vi "GenerateBurst.vi"(8 "error in (no error)":errorcluster, 9 "Burst mode":T1, 11 "reference in":refnum<class "niMmWave_Reciever.lvclass">) -> (0 "error out":errorcluster, 3 "reference out":refnum<class "niMmWave_Reciever.lvclass">)   [LabVIEW 2019, in "niMmWave_Reciever.lvclass"]
doc: "Generates single burst"
uses:
  niMmWave_Reciever.lvclass
  C:/Barkhausen mmWave radar/Development/LV/Barkhausen mmWave hardware control/Host/SubVIs/mmWave instrument_class/mmWave instrument.lvclass
  mmWave instrument_class/BurstMode.ctl
  mmWave HW Control/HW custom error.ctl
  mmWave instrument_class/Instrument state.ctl
  Low-level/TypeDefs/Direction.ctl
  mmWave HW Control/mmWave HW Control.lvlib
  mmWave instrument_class/mmWave instrument.lvclass
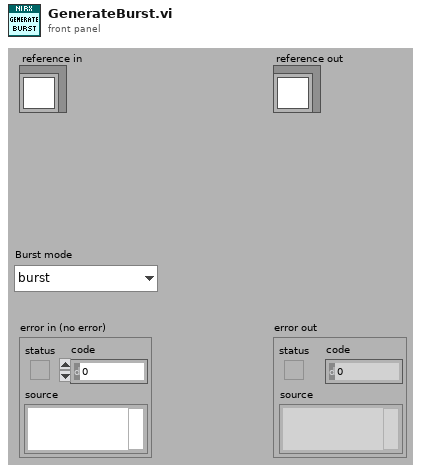
[diagram p1: front panel]
types:
  T1 = typedef "mmWave instrument.lvclass/BurstMode.ctl" = enum16{"burst", "continuous"}
  T2 = typedef "mmWave instrument.lvclass/Instrument state.ctl" = enum16{"Off", "Initialization", "Configuration", "Running", "Calibration"}
  T3 = typedef "Direction.ctl" = enum16{"Transceiver", "Receiver", "Transmitter"}
  T4 = typedef "mmWave HW Control.lvlib/HW custom error.ctl" = u16
  T5 = typedef "niMmWave_Reciever.lvclass/ObjectAttributesRef.ctl" = refnum<data-value>
  T6 = typedef "niMmWave_Reciever.lvclass/ObjectAttributes.ctl" = cluster{"session":T7[], "HW.RX devices":T20, "RF config":T21, "RX trigger options":T22, "RX samples":i32, "RX Fs":dbl}
  T7 = typedef "Session.ctl" = cluster{"3620 session":refnum<queue>, "tx baseband session":T8, "rx baseband session":T16, "tx gain (dB)":dbl, "rx gain (dB)":dbl, "hardware configuration":T17, "gain ranging":T18[], "pxi trigger bus information":T19}
  T8 = typedef "Tx Baseband Session.ctl" = cluster{"3610 session":T9, "7902 reference":T15}
  T9 = typedef "ni3610_and_ni3630_Driver_Lib.lvlib/Main Settings.ctl" = cluster{"VISA resource name":refnum<visa-resource-name>, "Address Space":T10, "window_offset":u32, "register_addresses":T11, "required_MM_fpga_version":cluster{"signature":u32, "hardware":u32, "current revision":u32, "oldest revision":u32}, "CPLD Oldest Compat Version ":cluster{"hardware":u32, "CPLD firmware":u32}, "MM_FPGA_image_location":string, "is_init":bool, "card_type":T12, "DacLmkConfigFileName":string, "AdcLmkConfigFileName":string, "AdcConfigFileName":string, "DacConfigFileName_RevA":string, "DacConfigFileName_RevB":string, "Mulde hardware revision":u8, "bypass DAC PLL\n":bool, "IQ Card Revision":T13, "board capability":T14}
  T10 = typedef "VISA Register Access Address Space.ctl" = u16
  T11 = typedef "ni3610_and_ni3630_Driver_Lib.lvlib/Register Adresses.ctl" = cluster{"MM based Registers":cluster{"Revision":u32, "OldestCompatRev":u32, "signature":u32, "scratch":u32, "LedControl":u32, "BoardHwRev":u32, "BoardControl":u32, "ThermalStatus":u32, "BasebandStatus":u32, "BasebandControl":u32, "BasebandAuxSetup":u32, "BasebandAuxStatus":u32, "LmkSyncOutSetup":u32, " AdcSyncOutSetup":u32, " InjSyncOutSetup":u32, " PxiTrig0OutSetup":u32, " PxiTrig1OutSetup":u32, " PxiTrig2OutSetup":u32, " PxiTrig3OutSetup":u32, " PxiTrig4OutSetup":u32, " PxiTrig5OutSetup":u32, " PxiTrig6OutSetup":u32, " PxiTrig7OutSetup":u32}, "CPLD based Registers":cluster{"SlaveSignature":u32, "SlaveRevision":u32, "SlaveOldestCompatRev":u32, "SlaveScratch":u32, "SlaveSetup":u32, "SlaveStatus":u32, "IDacReg_offset":u32, "LMKRegGrp0_offset":u32, "QDacReg_offset":u32, "BrdTempSensorVal":u32, "TempSensorPowerDown":u32, "GPIOReg_offset":u32, "IAdcReg_offset":u32, "QAdcReg_offset":u32, "LMKRegGrp1_offset":u32, "QadcTempSensorVal":u32, "IadcTempSensorVal":u32, "RevisionReg":u32, "VcxoReg":u32, "CpldStatusReg":u32, "PowerReg":u32, "VBiasEnReg":u32, "ExtRefOeReg":u32, "QdacCtrlReg":u32, "QdacStatusReg":u32, "IdacCtrlReg":u32, "IdacStatusReg":u32, "QdacJtagIn":u32, "QdacJtagOut":u32, "IdacJtagIn":u32, "IdacJtagOut":u32, "IqDcSetupReg":u32, "QadcStatusReg":u32, "IadcStatusReg":u32, "BrdSetupReg":u32, "IqDcRevisionReg":u32, "PllStatusReg":u32, "EndpointScratchReg":u32, "AdcSyncCfgReg":u32, "IqCardOpampReg":u32}, "CPLD Register Offset":u32, "MM  Register Offset":u32, " PxiTrig0OutSetup":u32}
  T12 = typedef "ni3610_and_ni3630_Driver_Lib.lvlib/Base Card Type.ctl" = enum16{"unspecified", "ADC", "DAC"}
  T13 = typedef "ni3610_and_ni3630_Driver_Lib.lvlib/IQ Card Revision.ctl" = enum16{"RevA", "RevB", "RevC", "RevD"}
  T14 = typedef "ni3610_and_ni3630_Driver_Lib.lvlib/Board Capability.ctl" = cluster{"baseband sync":enum16{"no baseband sync", "baseband sync"}}
  T15 = typedef "Blank FPGA Reference.ctl" = refnum<k20>
  T16 = typedef "Rx Baseband Session.ctl" = cluster{"3630 session":T9, "7902 reference":T15}
  T17 = typedef "Hardware Configuration.ctl" = cluster{"direction":T3, "baseband only":bool}
  T18 = typedef "Gain Ranging.ctl" = cluster{"gain ranging active scope":string, "gain ranging stream session":refnum<k20>}
  T19 = typedef "PXI Trigger Bus Info.ctl" = cluster{"chassis resource name":refnum<visa-resource-name>, "7902R (TX)":i16, "3610 (TX)":i16, "3620 (IF)":i16, "3630 (RX)":i16, "7902R (RX)":i16}
  T20 = typedef "mmWave HW Control.lvlib/HW RX resources cluster.ctl" = cluster{"HW.IF":tag, "HW.ADC":refnum<visa-resource-name>, "HW.RX FPGA":tag}
  T21 = typedef "mmWave HW Control.lvlib/HW RX RF config cluster.ctl" = cluster{"Gain":dbl, "Frequency":dbl, "mmWave adapter":string}
  T22 = typedef "TX trigger config.ctl" = cluster{"delay":dbl, "trig source":T23, "PXI src":i32, "export":T24, "PXI dest":i32}
  T23 = typedef "FPGA Utility.lvlib/FPGA driver trigger source.ctl" = enum16{"Use Tclk", "PXI_Trig", "Aurora RX trig"}
  T24 = typedef "FPGA Utility.lvlib/FPGA driver trigger destination.ctl" = enum16{"None", "Source trig", "Synced trig", "Delayed sync"}
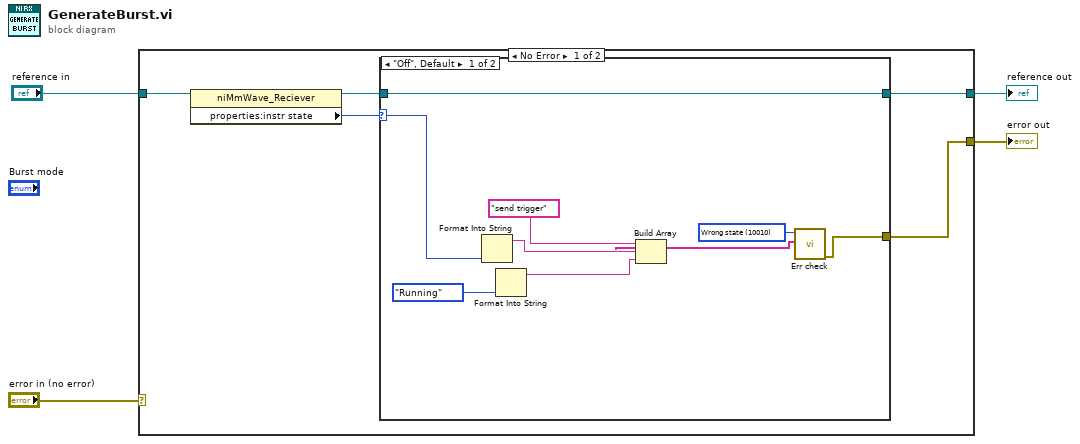
[diagram p0: block diagram]
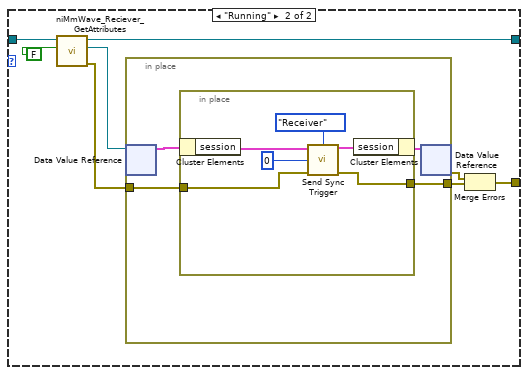
[diagram p2: hidden frame]
diagram:
  n1 = case shown="No Error" "error in (no error)" {
    selector: "error in (no error)" -> [_ w38]
    tunnel: [w7 w38] -> w3
    tunnel: [w8 w37] -> w1
    tunnel: "reference in" -> [w9 w37]
    frame No Error {
      n2 = property class="niMmWave_Reciever"(reference=w9) -> (reference out=w6:refnum<class "niMmWave_Reciever.lvclass">, "properties:instr state"=w5:T2)  [unwired: 1 in, 1 out]
      n3 = case shown="\"Off\", Default" w5 {
        selector: w5 -> [w10 _]
        tunnel: [w18 w26] -> w8
        tunnel: [w11 w20] -> w7
        tunnel: w6 -> [w18 w19]
        frame "Off", Default {
          w17 = T4 10010 items=["TX list"=10000, "TX length"=10001, "RX length"=10002, "Fs"=10003, "RF Fc"=10004, "Wrong state"=10010] ("HW custom err")
          n4 = Format Into String(w10) -> (resulting string=w15:string)  [unwired: 3 in, 1 out]
          n5 = Format Into String(Instrument_state."Running" ("properties:instr state")) -> (resulting string=w12:string)  [unwired: 3 in, 1 out]
          n6 = Build Array("send trigger", w15, w12) -> (w14:string[])
          n7 = call "Err check.vi"("Variant Control"=w14, "HW custom err"=w17) -> ("error out"=w11:errorcluster)  [unwired: 9 in]
        }
        frame "Running" {
          n8 = call "niMmWave_Reciever_GetAttributes.vi"("return data? (T)"=FALSE, "reference in"=w19) -> ("error out"=w23:errorcluster, "attributes ref"=w24:T5, "reference out"=w26:refnum<class "niMmWave_Reciever.lvclass">)  [unwired: 6 in, 1 out]
          n9 = in-place {
            in-place-border: w23 -> [w29]
            in-place-border: [w27] -> w22
            n10 = in-place-dvr #1(w24) -> (w30:T6)  [unwired: 1 out]
            n11 = in-place {
              in-place-border: w29 -> [w32]
              in-place-border: [w31] -> w27
              n12 = in-place-cluster #2(w30) -> ("session"=w34:T7[])
              n13 = call "Send Sync Trigger.vi"("session in"=w34, "sync select"=Direction."Receiver", "master device index"=0, "error in"=w32) -> ("session out"=w33:T7[], "error out"=w31:errorcluster)  [unwired: 10 in]
              n14 = in-place-cluster #2("session"=w33) -> (w28:T6)
            }
            n15 = in-place-dvr #1(w28) -> (w21:errorcluster)  [unwired: 1 out]
          }
          n16 = Merge Errors(w21, w22) -> (w20:errorcluster)
        }
      }
    }
    frame Error {
    }
  }
  "error out" <- w3
  "reference out" <- w1
